vi "Arrange Displays.vi"(0 "Number of Displays":u8, 2 "Action":T1(ring), 7 "IMAQ Display Refs":refnum<vi>[](array[refnum]), 11 "Aspect Ratio (Width/Height)":dbl, 13 "Z Scale Refs":refnum<vi>[](array[refnum])) -> (4 "Number of Displays Out":u8, 15 "Aspect Ratio (Width/Height) Out":dbl)   [LabVIEW 2016]
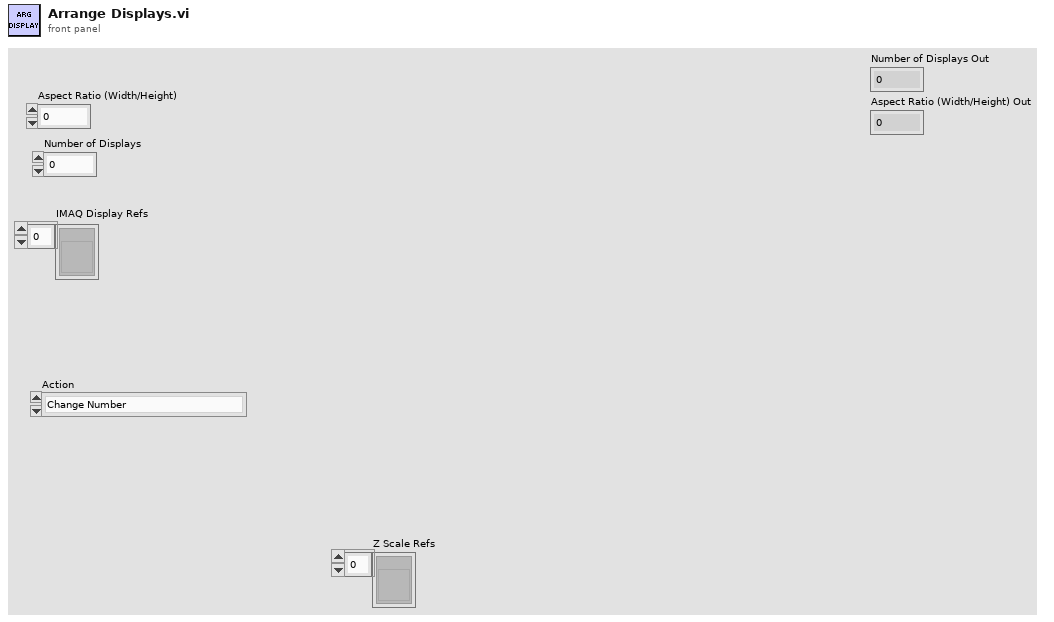
[diagram p1: front panel]
types:
  T1 = enum16{"Change Number", "Refresh Positions", "Get No. of Displays"}
  T2 = typedef "LVRectTypeDef.ctl" = cluster{"Left":i16, "Top":i16, "Right":i16, "Bottom":i16}
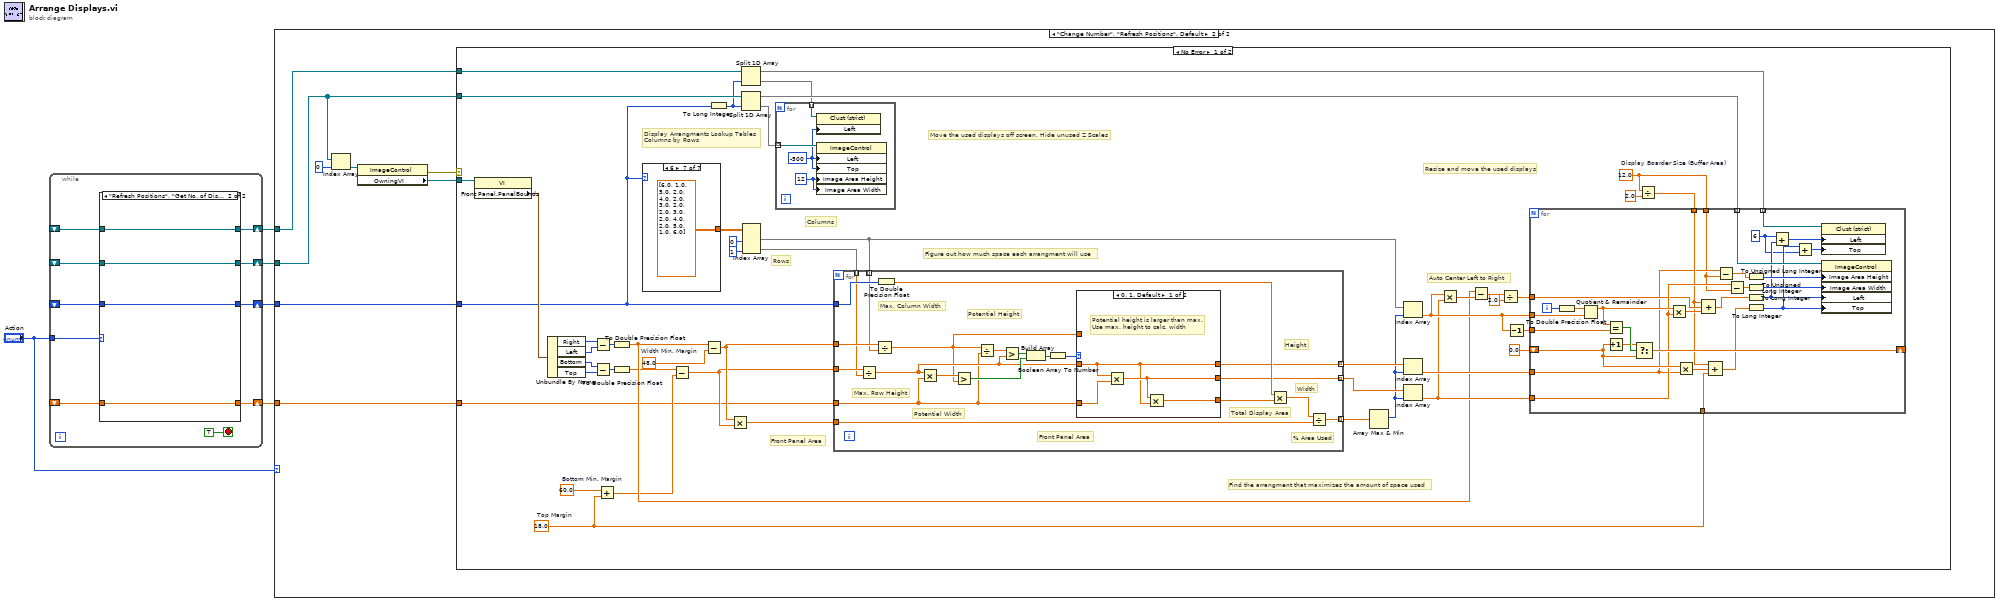
[diagram p0: block diagram]
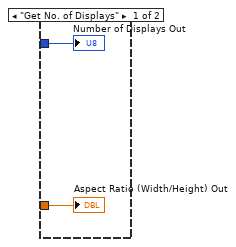
[diagram p2: hidden frame]
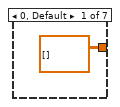
[diagram p3: hidden frame]
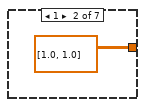
[diagram p4: hidden frame]
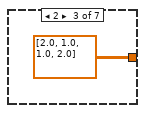
[diagram p5: hidden frame]
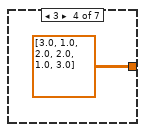
[diagram p6: hidden frame]
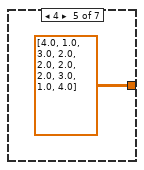
[diagram p7: hidden frame]
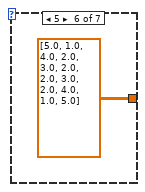
[diagram p8: hidden frame]
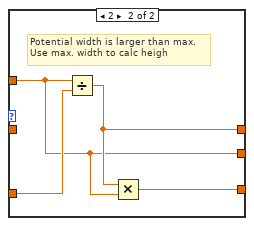
[diagram p9: hidden frame]
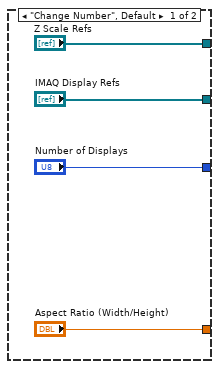
[diagram p11: hidden frame]
diagram:
  n1 = while {
    tunnel: "Action" -> [w14]
    shift-right: [w13] -> w5
    shift-left: _ -> [w11]
    shift-right: [w12] -> w4
    shift-left: _ -> [w10]
    shift-right: [w9] -> w3
    shift-left: _ -> [w8]
    shift-right: [w7] -> w1
    shift-left: _ -> [w6]
    stop <- TRUE stop-if-true
    n2 = case shown="\"Refresh Positions\", \"Get No. of Displays\"" w14 {
      tunnel: ["Aspect Ratio (Width/Height)" w22] -> w12
      tunnel: ["Number of Displays" w23] -> w13
      tunnel: w11 -> [_ w23]
      tunnel: w10 -> [_ w22]
      tunnel: ["IMAQ Display Refs" w21] -> w9
      tunnel: w8 -> [_ w21]
      tunnel: ["Z Scale Refs" w20] -> w7
      tunnel: w6 -> [_ w20]
      frame "Change Number", Default {
      }
      frame "Refresh Positions", "Get No. of Displays" {
      }
    }
  }
  n3 = case shown="\"Change Number\", \"Refresh Positions\", Default" "Action" {
    tunnel: w5 -> [w25 w30]
    tunnel: w4 -> [w24 w29]
    tunnel: w3 -> [_ w28]
    tunnel: w1 -> [_ w27]
    frame "Get No. of Displays" {
      "Number of Displays Out" <- w25
      "Aspect Ratio (Width/Height) Out" <- w24
    }
    frame "Change Number", "Refresh Positions", Default {
      n4 = Index Array(array=w28, index=0) -> (element=w32:refnum<vi>)
      n5 = property class="ImageControl"(reference=w32) -> (error out=w26:errorcluster, "OwningVI"=w31:refnum<vi>)  [unwired: 1 in, 1 out]
      n6 = case shown="No Error" w26 {
        tunnel: w31 -> [w45 _]
        tunnel: w30 -> [w40 _]
        tunnel: w29 -> [w39 _]
        tunnel: w28 -> [w38 _]
        tunnel: w27 -> [w37 _]
        frame No Error {
          w41 = 12.0  # Display Boarder Size (Buffer Area)
          w46 = 60.0  # Bottom Min. Margin
          w50 = 18.0  # Top Margin
          w59 = 48.0  # Width Min. Margin
          # "Auto Center Left to Right"
          # "Resize and move the used displays"
          # "Find the arrangment that maximizes the amount of space used"
          # "Figure out how much space each arrangment will use"
          # "Move the used displays off screen. Hide unused Z Scales"
          # "Front Panel Area"
          # "Rows"
          # "Columns"
          # "Display Arrangments Lookup Tables\nColumns by Rows"
          n7 = property class="VI"(reference=w45) -> ("Front Panel.PanelBounds"=w44:T2)  [unwired: 1 in, 2 out]
          n8 = Unbundle By Name(w44) -> ("Right"=w80:i16, "Left"=w79:i16, "Bottom"=w78:i16, "Top"=w77:i16)
          n9 = Subtract(x=w80, y=w79) -> (x-y=w76:i16)
          n10 = Subtract(x=w78, y=w77) -> (x-y=w75:i16)
          n11 = Add(x=w46, y=w50) -> (x+y=w49:dbl)
          n12 = To Double Precision Float(number=w76) -> (double precision float=w51:dbl)
          n13 = To Double Precision Float(number=w75) -> (double precision float=w48:dbl)
          n14 = case shown="6" w40 {
            tunnel: [dbl[][] [] dbl[][] [[1.0, 1.0]] dbl[][] [[2.0, 1.0], [1.0, 2.0]] dbl[][] [[3.0, 1.0], [2.0, 2.0], [1.0, 3.0]] dbl[][] [[4.0, 1.0], [3.0, 2.0], [2.0, 2.0], [2.0, 3.0], [1.0, 4.0]] dbl[][] [[5.0, 1.0], [4.0, 2.0], [3.0, 2.0], [2.0, 3.0], [2.0, 4.0], [1.0, 5.0]] dbl[][] [[6.0, 1.0], [5.0, 2.0], [4.0, 2.0], [3.0, 2.0], [2.0, 3.0], [2.0, 4.0], [2.0, 5.0], [1.0, 6.0]]] -> w73
            frame 0, Default {
            }
            frame 1 {
            }
            frame 2 {
            }
            frame 3 {
            }
            frame 4 {
            }
            frame 5 {
            }
            frame 6 {
            }
          }
          n15 = Subtract(x=w48, y=w49) -> (x-y=w47:dbl)
          n16 = Subtract(x=w51, y=w59) -> (x-y=w58:dbl)
          n17 = To Long Integer(number=w40) -> (32bit integer=w36:i32)
          n18 = Multiply(x=w58, y=w47) -> (x*y=w74:dbl)
          n19 = Split 1D Array(array=w37, index=w36) -> (first subarray=w34:refnum<vi>[], second subarray=w35:refnum<vi>[])
          n20 = Split 1D Array(array=w38, index=w36) -> (first subarray=w61:refnum<vi>[], second subarray=w60:refnum<vi>[])
          n21 = Index Array(array=w73, index (col) #1=0 ("disabled index (col)"), index (col) #2=1 ("index (col)")) -> (element #1=w66:dbl[], element #2=w65:dbl[])  [unwired: 2 in]
          n22 = for {
            tunnel: w60 -> [w84] mode=indexing
            tunnel: w35 -> [w82] mode=indexing
            w83 = u32 12 ("Image Area:Size:Height")
            w81 = -500 ("Position:Left")
            n23 = property class="Clust (strict)"(reference=w82, "Left"=w81) -> ()  [unwired: 1 in, 2 out]
            n24 = property class="ImageControl"(reference=w84, "Left"=w81, "Top"=w81, "Image Area Height"=w83, "Image Area Width"=w83) -> ()  [unwired: 1 in, 2 out]
          }
          n25 = for {
            tunnel: w39 -> [w133]
            tunnel: w58 -> [w142]
            tunnel: w47 -> [w141]
            tunnel: w74 -> [w127]
            tunnel: [w130] -> w69 mode=indexing
            tunnel: [w129] -> w68 mode=indexing
            tunnel: [w126] -> w70 mode=indexing
            tunnel: w66 -> [w123] mode=indexing
            tunnel: w65 -> [w122] mode=indexing
            tunnel: w40 -> [w124]
            # "% Area Used"
            # "Front Panel Area"
            # "Total Display Area"
            # "Width"
            # "Height"
            # "Potential Height"
            # "Potential Width"
            # "Max. Row Height"
            # "Max. Column Width"
            n26 = Divide(x=w141, y=w122) -> (x/y=w135:dbl)
            n27 = Divide(x=w142, y=w123) -> (x/y=w134:dbl)
            n28 = To Double Precision Float(number=w124) -> (double precision float=w131:dbl)
            n29 = Multiply(x=w135, y=w133) -> (x*y=w140:dbl)
            n30 = Greater?(x=w140, y=w134) -> (0:w137:bool)
            n31 = Divide(x=w134, y=w133) -> (x/y=w139:dbl)
            n32 = Greater?(x=w139, y=w135) -> (0:w138:bool)
            n33 = Build Array(w138, w137) -> (w136:bool[])
            n34 = Boolean Array To Number(Boolean array=w136) -> (number=w125:u32)
            n35 = case shown="0, 1, Default" w125 {
              tunnel: w135 -> [w144 _]
              tunnel: w134 -> [_ w148]
              tunnel: w133 -> [w146 w150]
              tunnel: [w144 w149] -> w130
              tunnel: [w145 w148] -> w129
              tunnel: [w143 w147] -> w132
              frame 0, 1, Default {
                # "Potential height is larger than max.\nUse max. height to calc. width"
                n36 = Multiply(x=w144, y=w146) -> (x*y=w145:dbl)
                n37 = Multiply(x=w145, y=w144) -> (x*y=w143:dbl)
              }
              frame 2 {
                # "Potential width is larger than max.\nUse max. width to calc heigh"
                n38 = Divide(x=w148, y=w150) -> (x/y=w149:dbl)
                n39 = Multiply(x=w149, y=w148) -> (x*y=w147:dbl)
              }
            }
            n40 = Multiply(x=w131, y=w132) -> (x*y=w128:dbl)
            n41 = Divide(x=w128, y=w127) -> (x/y=w126:dbl)
          }
          n42 = Array Max & Min(array=w70) -> (max index (indices)=w64:i32)  [unwired: 3 out]
          n43 = Index Array(array=w66, index=w64) -> (element=w57:dbl)
          n44 = Index Array(array=w69, index=w64) -> (element=w67:dbl)
          n45 = Index Array(array=w68, index=w64) -> (element=w56:dbl)
          n46 = Multiply(x=w57, y=w56) -> (x*y=w55:dbl)
          n47 = Subtract(x=w51, y=w55) -> (x-y=w54:dbl)
          n48 = Divide(x=w54, y=2.0) -> (x/y=w52:dbl)
          n49 = Decrement(x=w57) -> (x-1=w63:dbl)
          n50 = Divide(x=w41, y=2.0) -> (x/y=w42:dbl)
          n51 = for {
            tunnel: w67 -> [w93]
            tunnel: w56 -> [w102]
            tunnel: w57 -> [w114]
            tunnel: w61 -> [w105] mode=indexing
            tunnel: w63 -> [w111]
            shift-right: [w108] -> _
            shift-left: 0.0 -> [w107]
            tunnel: w52 -> [w98]
            tunnel: w50 -> [w97]
            tunnel: w42 -> [w94]
            tunnel: w41 -> [w92]
            tunnel: w34 -> [w90] mode=indexing
            i -> [w112]
            w85 = 6 ("x")
            n52 = To Double Precision Float(number=w112) -> (double precision float=w113:dbl)
            n53 = Quotient & Remainder(x=w113, y=w114) -> (x-y*floor(x/y)=w106:dbl)  [unwired: 1 out]
            n54 = Equal?(x=w106, y=w111) -> (x = y?=w110:bool)
            n55 = Increment(x=w107) -> (x+1=w109:dbl)
            n56 = Select(t=w109, s=w110, f=w107) -> (s? t:f=w108:dbl)
            n57 = Multiply(x=w106, y=w102) -> (x*y=w100:dbl)
            n58 = Multiply(x=w107, y=w93) -> (x*y=w96:dbl)
            n59 = Compound Arithmetic op=ADD(w94, w98, w100) -> (w99:dbl)
            n60 = Compound Arithmetic op=ADD(w94, w96, w97) -> (w95:dbl)
            n61 = Subtract(x=w93, y=w92) -> (x-y=w91:dbl)
            n62 = Subtract(x=w102, y=w92) -> (x-y=w101:dbl)
            n63 = To Unsigned Long Integer(number=w91) -> (unsigned 32bit integer=w104:u32)
            n64 = To Unsigned Long Integer(number=w101) -> (unsigned 32bit integer=w103:u32)
            n65 = To Long Integer(number=w99) -> (32bit integer=w89:i32)
            n66 = To Long Integer(number=w95) -> (32bit integer=w86:i32)
            n67 = Add(x=w85, y=w89) -> (x+y=w88:i32)
            n68 = Add(x=w86, y=w85) -> (x+y=w87:i32)
            n69 = property class="Clust (strict)"(reference=w90, "Left"=w88, "Top"=w87) -> ()  [unwired: 1 in, 2 out]
            n70 = property class="ImageControl"(reference=w105, "Image Area Height"=w104, "Image Area Width"=w103, "Left"=w89, "Top"=w86) -> ()  [unwired: 1 in, 2 out]
          }
        }
        frame Error {
        }
      }
    }
  }
